vi "Read SCPI Error Queue (GPIB).vi"(2 "error in":T1, 3 "GPIB address":string) -> (0 "error out":T1, 1 "messages":string)   [LabVIEW 2019]
doc: "This VI reads the status message from the power meter and determines whether an error has occurred during the previous operations. If an error is detected, the front panel LED (error) will be turned on, and the messages will be displayed."
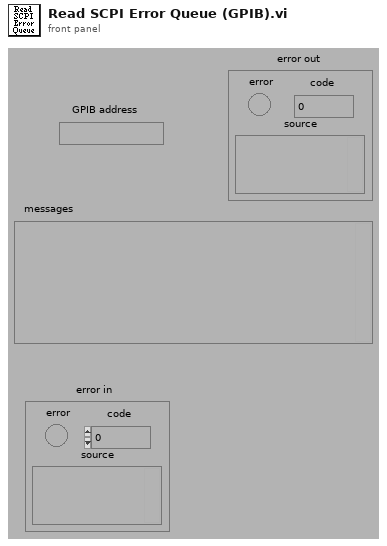
[diagram p1: front panel]
types:
  T1 = cluster{"error":bool, "code":i32, "source":string}
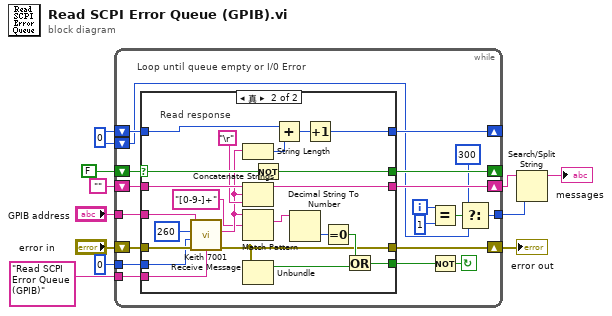
[diagram p0: block diagram]
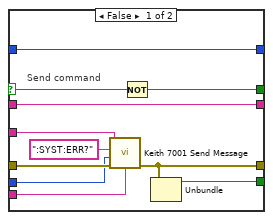
[diagram p2: hidden frame]
diagram:
  w7 = 0
  n1 = while {
    tunnel: [w16] -> w4
    shift-left: w7 -> [w17]
    shift-left: w7 -> [w19]
    shift-right: [w18] -> _
    tunnel: 0 -> [w20]
    tunnel: "Read SCPI Error Queue (GPIB)" -> [w21]
    shift-left: "error in" -> [w23]
    shift-right: [w22] -> w1
    tunnel: "GPIB address" -> [w24]
    shift-left: FALSE -> [w26]
    shift-right: [w25] -> _
    shift-left: "" -> [w29]
    shift-right: [w30] -> w6
    i -> [w15]
    stop <- w27 continue-if-true
    # "Loop until queue empty or I/0 Error"
    n2 = case shown="真" w26 {
      selector: w26 -> [w40 w59]
      tunnel: [w36 w62] -> w28
      tunnel: [w41 w61] -> w30
      tunnel: w29 -> [w41 w60]
      tunnel: [w39 w58] -> w25
      tunnel: w24 -> [w37 w54]
      tunnel: [w33 w53] -> w22
      tunnel: w23 -> [w35 w51]
      tunnel: w21 -> [w34 w49]
      tunnel: w20 -> [w32 w50]
      tunnel: w19 -> [w31 w47]
      tunnel: [w31 w45] -> w18
      frame False {
        # "Send command"
        n3 = call "Keith 7001 Send Message.vi"("address string"=w37, "write buffer"=":SYST:ERR?", "source"=w34, "write mode (set END:0)"=w32, "error in"=w35) -> ("error out"=w33:T1)  [unwired: 1 in, 3 out]
        n4 = Not(x=w40) -> (.not. x?=w39:bool)
        n5 = Unbundle(w33) -> ("error"=w36:bool)  [unwired: 2 out]
      }
      frame True {
        # "Read response"
        n6 = call "Keith 7001 Receive Message.vi"("address string"=w54, "byte count"=260, "source"=w49, "read mode"=w50, "error in"=w51) -> ("read buffer"=w44:string, "error out"=w53:T1)  [unwired: 1 in, 2 out]
        n7 = String Length(string=w44) -> (length=w48:i32)
        n8 = Concatenate Strings(w60, w44, "\r") -> (w61:string)
        n9 = Match Pattern(string=w44, regular expression="[0-9-]+") -> (match substring=w42:string)  [unwired: 1 in, 3 out]
        n10 = Unbundle(w53) -> ("error"=w52:bool)  [unwired: 2 out]
        n11 = Not(x=w59) -> (.not. x?=w58:bool)
        n12 = Add(x=w47, y=w48) -> (x+y=w46:i32)
        n13 = Decimal String To Number(string=w42) -> (number=w63:i32)  [unwired: 2 in, 1 out]
        n14 = Increment(x=w46) -> (x+1=w45:i32)
        n15 = Equal To 0?(x=w63) -> (x = 0?=w57:bool)
        n16 = Or(x=w57, y=w52) -> (x .or. y?=w62:bool)
      }
    }
    n17 = Equal?(x=w15, y=1) -> (x = y?=w13:bool)
    n18 = Not(x=w28) -> (.not. x?=w27:bool)
    n19 = Select(t=300, s=w13, f=w17) -> (s? t:f=w16:i32)
  }
  "error out" <- w1
  n20 = Search/Split String(string=w6, offset (0)=w4) -> (substring before match=→"messages":string)  [unwired: 1 in, 2 out]
